vi "Declare_Sync_Client.vi"   [LabVIEW 2010]
uses:
  ADAM Client/Sub VIs/ADAM Controls/Channel_State.ctl
  ADAM Client/Sub VIs/ADAM Controls/Ch_description_ADAM.ctl
  ADAM Client/Sub VIs/ADAM Controls/Module_type_ADAM.ctl
  ADAM Client/Sub VIs/ADAM Controls/Function_ADAM.ctl
  ADAM Client/Sub VIs/ADAM Controls/Calib_type_ADAM.ctl
  ADAM Client/Sub VIs/ADAM Controls/Address.ctl
  ADAM Client/Sub VIs/ADAM Controls/Update_scan_value.ctl
  Globals/Preference_global.vi
types:
  T1 = typedef "Channel_State.ctl" = enum16{"On", "Off", "Always On", "Always Off"}
  T2 = typedef "Ch_description_ADAM.ctl" = cluster{"Ch Name":string, "Type":T3, "Function":T4, "Ch State":T1, "Calibration type":T5, "A":dbl, "B":dbl, "C":dbl, "D":dbl, "Comments":string, "Address":T6, "String":string, "Duty":u16}
  T3 = typedef "Module_type_ADAM.ctl" = enum16{"4011", "4012", "4013", "4014", "4016", "4017", "4018", "4021", "4050", "4052", "4053", "4060", "4080", "5000", "5017", "5018", "5024", "5051", "5056", "5060", "6060", "Tracker", "WEST", "GILL", "JEM", "VICI", "Vaisala", "DRUCK", "Run VI Named:", "IR2100", "PPT", "Comparator", "VIRTUAL", "Hold Value", "Read A", "Read Ch", "Coded", "Client Info", "Web Client", "X10", "Test"}
  T4 = typedef "Function_ADAM.ctl" = enum16{"Analogue Input", "Digital Input", "Event counter", "Event rate", "Analogue Output", "Digital Output", "Relay Output"}
  T5 = typedef "Calib_type_ADAM.ctl" = enum16{"Raw", "Bx + A", "Cx^2 + Bx + A", "Dx^3 + Cx^2 + Bx + A", "In Band", "Hi-Tec Q", "Hi-Tec M_dot", "Text"}
  T6 = typedef "Address.ctl" = cluster{"Main":i32, "Ch.":i32, "Sub":i32, "Port Name":string}
  T7 = typedef "Update_scan_value.ctl" = cluster{"Channel Name":string, "New Value":dbl}
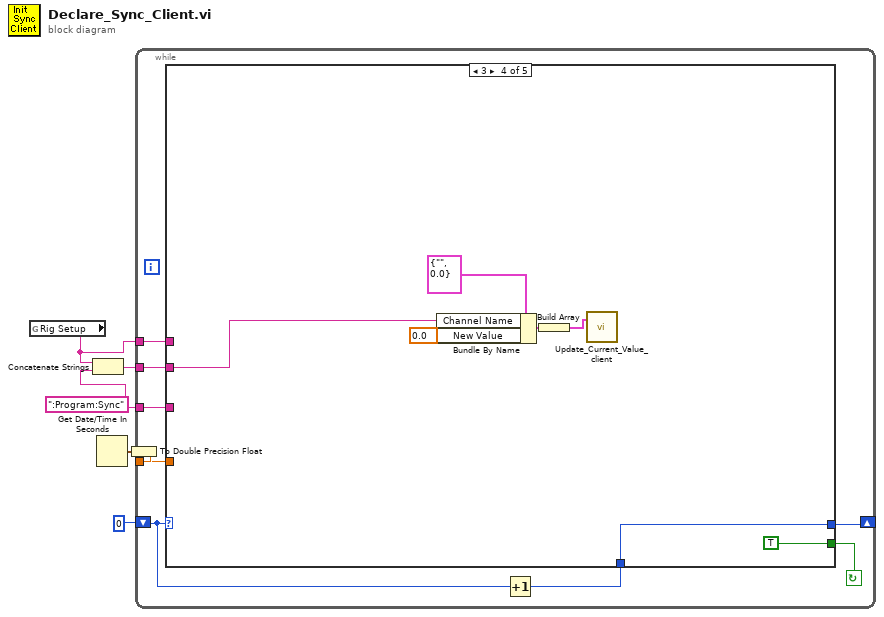
[diagram p0: block diagram]
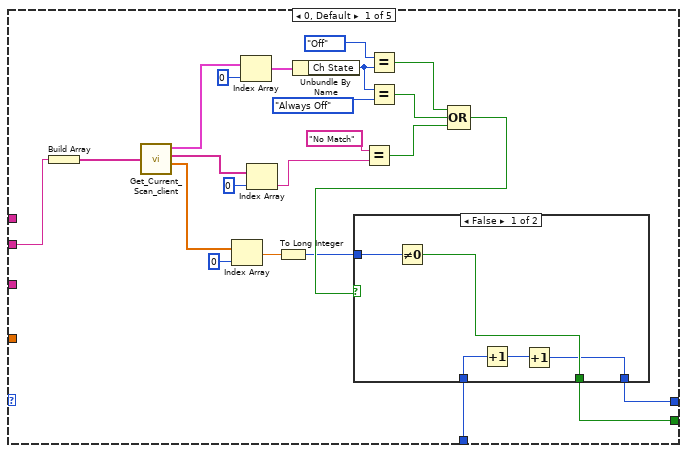
[diagram p2: hidden frame]
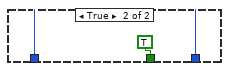
[diagram p3: hidden frame]
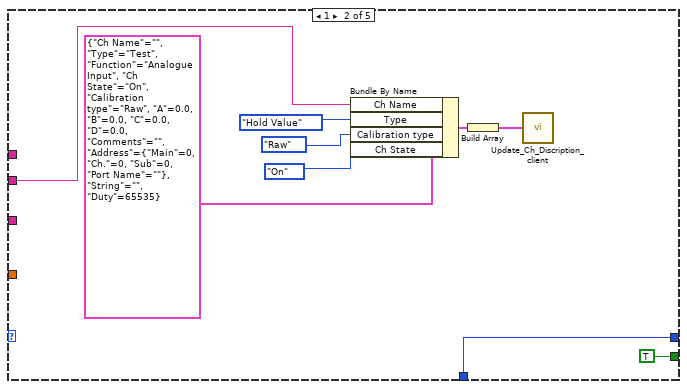
[diagram p4: hidden frame]
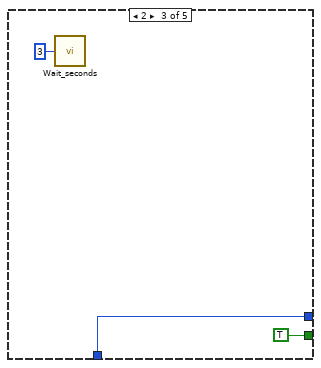
[diagram p5: hidden frame]
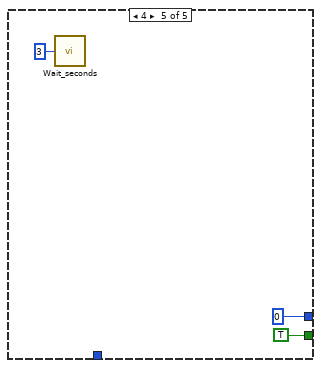
[diagram p6: hidden frame]
diagram:
  w5 = ":Program:Sync"
  n1 = global read "Preference_global.vi" "Rig Setup"() -> (w2:string)
  n2 = Concatenate Strings(w2, w5) -> (w4:string)
  n3 = Get Date/Time In Seconds() -> (seconds since 1Jan1904=w1:timestamp)
  n4 = To Double Precision Float(number=w1) -> (double precision float=w6:dbl)
  n5 = while {
    tunnel: w2 -> [w7]
    tunnel: w6 -> [w8]
    tunnel: w4 -> [w9]
    tunnel: w5 -> [w10]
    shift-left: 0 -> [w13]
    shift-right: [w12] -> _
    stop <- w14 continue-if-true
    n6 = Increment(x=w13) -> (x+1=w11:i32)
    n7 = case shown="3" w13 {
      tunnel: [w15 TRUE TRUE TRUE TRUE] -> w14
      tunnel: [w20 w45 w56 w57 0] -> w12
      tunnel: w11 -> [w21 w45 w56 w57 _]
      tunnel: w10 -> [_ _ _ _ _]
      tunnel: w9 -> [w23 w46 _ w59 _]
      tunnel: w8 -> [_ _ _ _ _]
      tunnel: w7 -> [_ _ _ _ _]
      frame 0, Default {
        n8 = Build Array(w23) -> (w24:string[])
        n9 = call "Get_Current_Scan_client.vi"("ADAM Ch Names"=w24) -> ("Ch Description Array"=w32:T2[], "String values"=w35:string[], "Numerical Values"=w18:dbl[])  [unwired: 1 out]
        n10 = Index Array(array=w18, index=0 ("Index")) -> (element=w17:dbl)
        n11 = Index Array(array=w32, index=0 ("Index")) -> (element=w31:T2)
        n12 = Index Array(array=w35, index=0 ("Index")) -> (element=w34:string)
        n13 = To Long Integer(number=w17) -> (32bit integer=w16:i32)
        n14 = Unbundle By Name(w31) -> ("Ch State"=w29:T1)
        n15 = Equal?(x="No Match", y=w34) -> (x = y?=w25:bool)
        n16 = Equal?(x=Channel_State."Off" ("Ch State"), y=w29) -> (x = y?=w27:bool)
        n17 = Equal?(x=w29, y=Channel_State."Always Off" ("Ch State")) -> (x = y?=w26:bool)
        n18 = Compound Arithmetic op=OR(w27, w26, w25) -> (w22:bool)
        n19 = case shown="False" w22 {
          tunnel: w21 -> [w40 w44]
          tunnel: [w38 w44] -> w20
          tunnel: w16 -> [w42 _]
          tunnel: [w41 TRUE] -> w15
          frame False {
            n20 = Not Equal To 0?(x=w42) -> (x != 0?=w41:bool)
            n21 = Increment(x=w40) -> (x+1=w39:i32)
            n22 = Increment(x=w39) -> (x+1=w38:i32)
          }
          frame True {
          }
        }
      }
      frame 1 {
        n23 = Bundle By Name(cluster=T2 {"Ch Name"="", "Type"=enum."Test", "Function"=enum."Analogue Input", "Ch State"=enum."On", "Calibration type"=enum."Raw", "A"=0.0, "B"=0.0, "C"=0.0, "D"=0.0, "Comments"="", "Address"={"Main"=0, "Ch."=0, "Sub"=0, "Port Name"=""}, "String"="", "Duty"=65535} ("Ch Discription"), "Ch Name"=w46, "Type"=Module_type_ADAM."Hold Value", "Calibration type"=Calib_type_ADAM."Raw", "Ch State"=Channel_State."On") -> (w52:T2)
        n24 = Build Array(w52) -> (w53:T2[])
        n25 = call "Update_Ch_Discription_client.vi"("Channels to update In"=w53) -> ()  [unwired: 1 out]
      }
      frame 2 {
        n26 = call "Wait_seconds.vi"("Seconds to wait"=u32 3) -> ()
      }
      frame 3 {
        n27 = Bundle By Name(cluster=T7 {"Channel Name"="", "New Value"=0.0} ("Update Scan Value Cluster"), "Channel Name"=w59, "New Value"=0.0 ("Bundle Element")) -> (w62:T7)
        n28 = Build Array(w62) -> (w60:T7[])
        n29 = call "Update_Current_Value_client.vi"("Update array in"=w60) -> ()  [unwired: 1 in]
      }
      frame 4 {
        n30 = call "Wait_seconds.vi"("Seconds to wait"=u32 3) -> ()
      }
    }
  }
